vi "PS35_GetErrorState.vi"(3 "error in (no error)":errorcluster, 4 "Axis number":i32=1 min=0 max=3, 5 "Control unit ID":i32=1 min=1 max=10) -> (0 "error out":errorcluster, 1 "Error state":i32)   [LabVIEW 2020]
doc: "PS35_GetErrorState.vi, created: 04.03.2009 alex; last change: 22.10.2019 alex;\n\n<B>FUNCTION:</B> \n\nRead error state.\nWith this function it is determined whether an axis was switched off\nor stopped because of an error while positioning.\n----------------------------------------------------------------------------------------\n<B>INPUT:</B>\n[I32] <B>Control unit ID:</B> control unit index. (Default=1, Range=1...10) \n[I32] <B>Axis number:</B> axis number. (Default=1, Range=0...3)\n0 - read state of all axes,\n1...3 - read state of an axis. \n[CLU] <B>error in</B>\n----------------------------------------------------------------------------------------\n<B>OUTPUT:</B>\n[I32] <B>Error state:</B> state of an axis or all axes.\nAxis number = 0 (all axes)\n0 - all axes are error-free and switched on,\n1 - all axes are error-free, any axis is switched off,\n2 - any axis is switched off or stopped because of an error.\nAxis number = 1...3 (an axis)\n0 - axis is error-free and switched on,\n1 - axis is error-free and switched off,\n2 - axis is switched off after an actuation of a limit switch,\n3 - axis is stopped after an actuation of a brake switch,\n4 - axis is switched off because of a power amplifier error,\n5 - axis is switched off because of a motion controller error,\n6 - axis is switched off because of a timeout error,\n7 - phases initialization is active (step motor axis),\n8 - axis is switched off because of a positioning error,\n9 - unknown axis error.\n[CLU] <B>error out</B>\n----------------------------------------------------------------------------------------\n<B>SUB-VIs:</B>\nPS35_GetReadError.vi\n----------------------------------------------------------------------------------------\n<B>EXT-Calls:</B>\nps35.dll (V2.01)\n----------------------------------------------------------------------------------------"
uses:
  ps35.dll
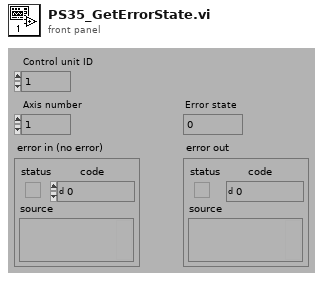
[diagram p1: front panel]
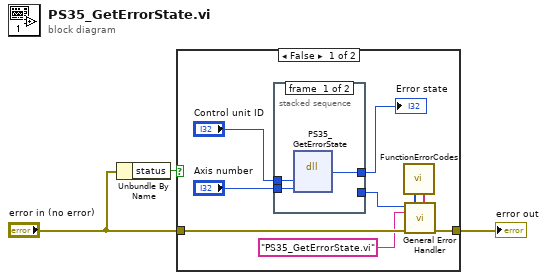
[diagram p0: block diagram]
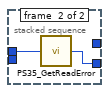
[diagram p2: hidden frame]
diagram:
  n1 = Unbundle By Name("error in (no error)") -> ("status"=w1:bool)
  n2 = case shown="False" w1 {
    tunnel: "error in (no error)" -> [w11 w18]
    tunnel: [w10 w18] -> w3
    frame False {
      n3 = stacked-sequence {
        tunnel: "Control unit ID" -> [w15 w17]
        tunnel: [w14 _] -> w9
        tunnel: [_ w16] -> w8
        tunnel: "Axis number" -> [w13 _]
        frame #0 {
          n4 = dll-call lib="C:/GEECS/Developers Version/source/Device Drivers/OwiSoft/OWISoftOEM/ps35/labview/lv82/ps35.dll" fn="PS35_GetErrorState" label="PS35_Get\nErrorState"("Index"=w15, "AxisNr"=w13) -> ("Rückgabetyp"=w14:i32)  [unwired: 5 in, 2 out]
        }
        frame #1 {
          n5 = call "PS35_GetReadError.vi"("Control unit ID"=w17) -> ("Read error"=w16:i32)
        }
      }
      "Error state" <- w9
      n6 = call "FunctionErrorCodes.vi"() -> ("[user-defined codes]"=w4:i32[], "[user-defined descriptions]"=w5:string[])  [unwired: 8 in]
      n7 = call <vilib>:"General Error Handler.vi"("[error code] (0)"=w8, "[user-defined codes]"=w4, "[user-defined descriptions]"=w5, "[error source] (\" \")"="PS35_GetErrorState.vi" ("[error source] (\" \")"), "error in (no error)"=w11) -> ("error out"=w10:errorcluster)  [unwired: 6 in, 4 out]
    }
    frame True {
    }
  }
  "error out" <- w3
